vi "getParameters.vi"(11 "TestHardpointCommand in":refnum<class "TestHardpointCommand.lvclass">) -> (2 "Parameters":T1, 3 "TestHardpointCommand out":refnum<class "TestHardpointCommand.lvclass">)   [LabVIEW 2016, in "TestHardpointCommand.lvclass"]
uses:
  TestHardpointCommand.lvclass
  DataTypes/Topics/CommandTestHardpoint.ctl
  DataTypes/Topics/Parts/CommandId.ctl
  TestHardpointCommand.lvclass/TestHardpointCommand.ctl
  DataTypes/Topics/M1M3SupportTopics.lvlib
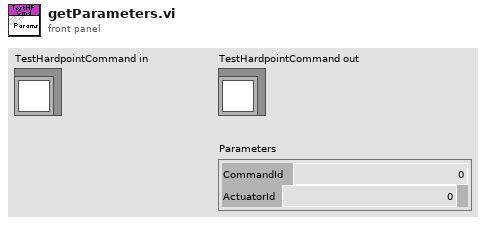
[diagram p1: front panel]
types:
  T1 = typedef "M1M3SupportTopics.lvlib/CommandTestHardpoint.ctl" = cluster{"CommandId":T2, "ActuatorId":i32}
  T2 = typedef "M1M3SupportTopics.lvlib/CommandId.ctl" = i32
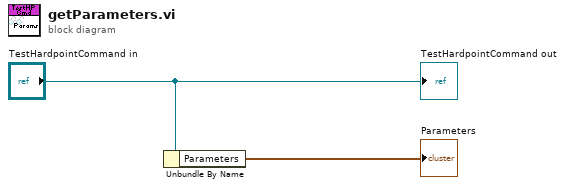
[diagram p0: block diagram]
diagram:
  n1 = Unbundle By Name("TestHardpointCommand in") -> ("Parameters"=→"Parameters":T1)
  "TestHardpointCommand out" <- "TestHardpointCommand in"
